vi "Dual_DM_Control_Main_V2.vi"(7 "Calling VI Ref":refnum<vi>) -> ()   [LabVIEW 2016]
uses:
  Controls/MirrorModes.ctl
  Hardware Configuration/Hardware Configuration Controls/Standard Action.ctl
  <vilib>/Utility/miscctls.llb/LVPointTypeDef.ctl
  <vilib>/Analysis/baseanly.llb/Mean (DBL).vi
  <vilib>/Utility/file.llb/Read Delimited Spreadsheet (DBL).vi
  <vilib>/Analysis/NI_AALBase.lvlib
  <vilib>/Utility/file.llb/Write To Spreadsheet File (DBL).vi
  <vilib>/Utility/file.llb/Read From Spreadsheet File (DBL).vi
panel:
  in  "Astig On/Off":bool
  in  "Load Astig":bool
  in  "Active Mirror":enum32{"Mirror 1", "Mirror 2"}(radio)
  in  "Clear Modes":bool
  in  "Mirror Modes":T1
  in  "Load Modes":bool
  in  "Save Modes":bool
  in  "Load Flat":bool
  in  "Apply Zero":bool
  in  "Load V Map":bool
  in  "Save V Map":bool
  in  "Apply Flat":bool
  in  "Center Bias":bool
  in  "Quit":bool
  out "Pixel Map (-1 to 1)":dbl[][](graph)
  # "Mode"
  # "Amount (nm)"
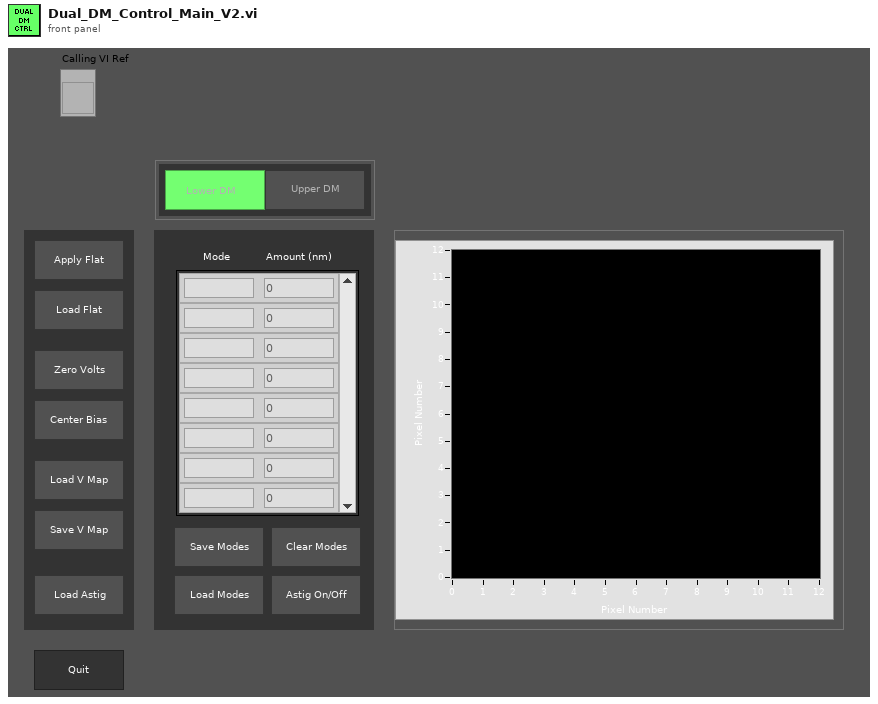
[diagram p1: front panel]
types:
  T1 = typedef "MirrorModes.ctl" = cluster{"Mode":string, "Amplitude":dbl}[]
  T2 = enum16{"Always On", "Always Off", "Off While Running"}
  T3 = typedef "LVPointTypeDef.ctl" = cluster{"Horizontal":i16, "Vertical":i16}
  T4 = typedef "Standard Action.ctl" = enum16{"Read", "Write"}
  T5 = typedef "MirrorModes_DUAL.ctl" = cluster{"Mode":string, "Amplitude":dbl}[][]
  T6 = typedef "LVRectTypeDef.ctl" = cluster{"Left":i16, "Top":i16, "Right":i16, "Bottom":i16}
  T7 = typedef "LVBoundsTypeDef.ctl" = cluster{"Width":u32, "Height":u32}
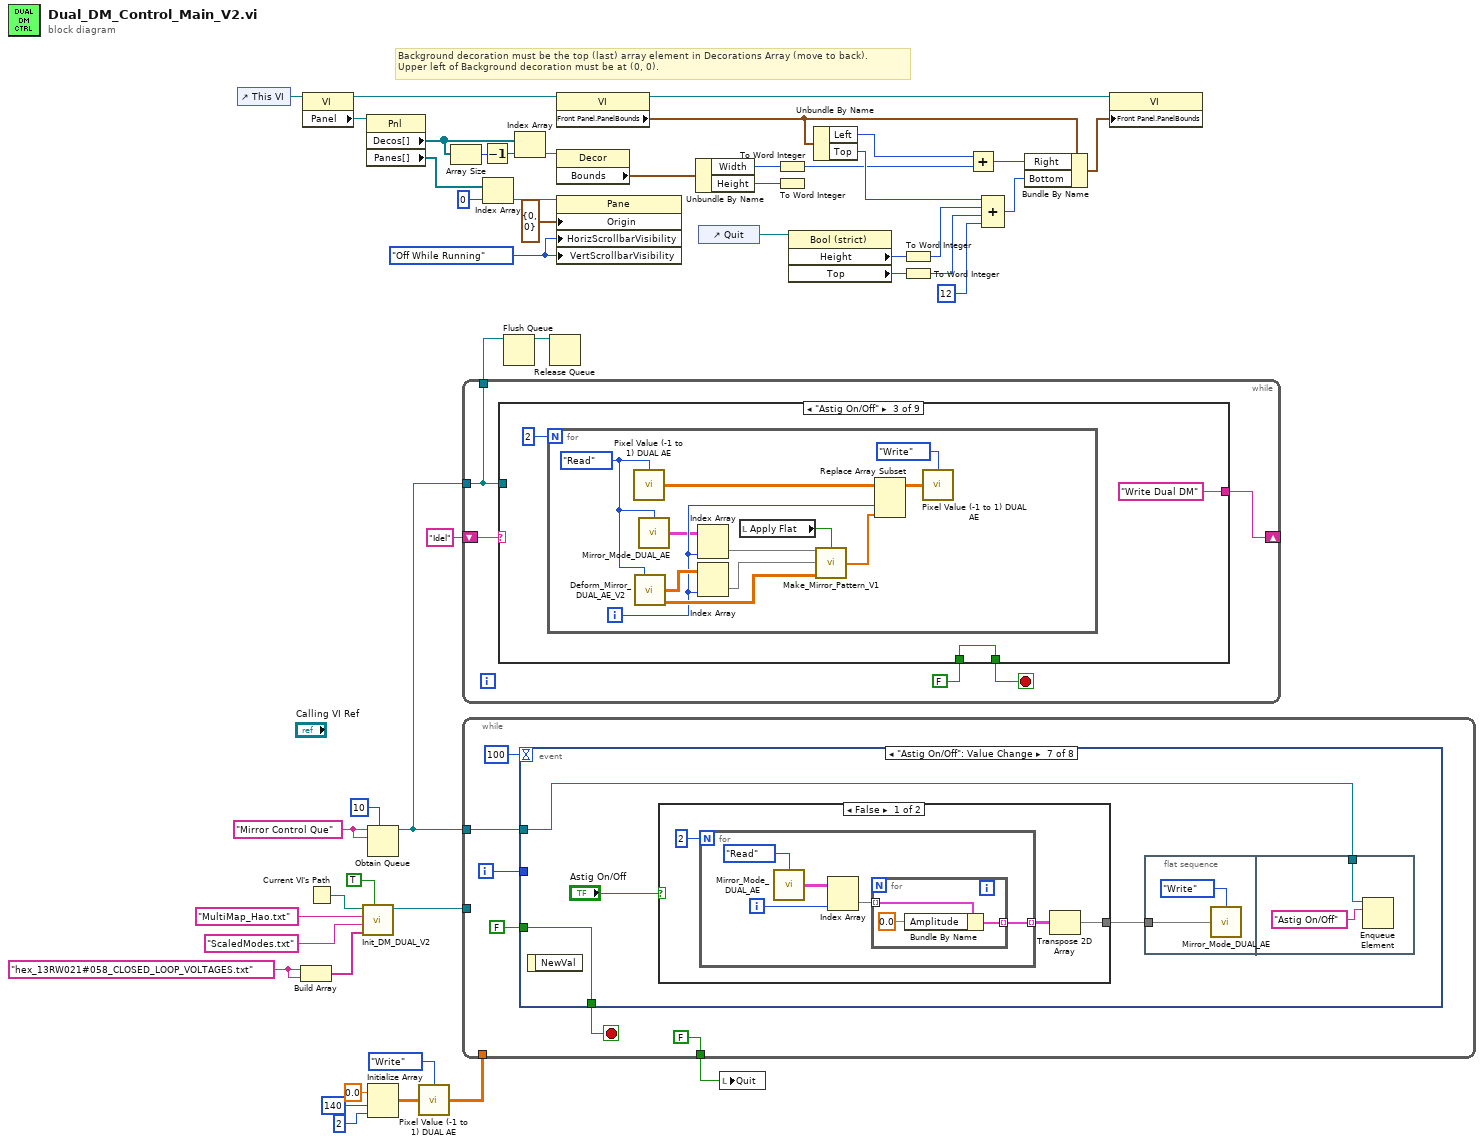
[diagram p0: block diagram]
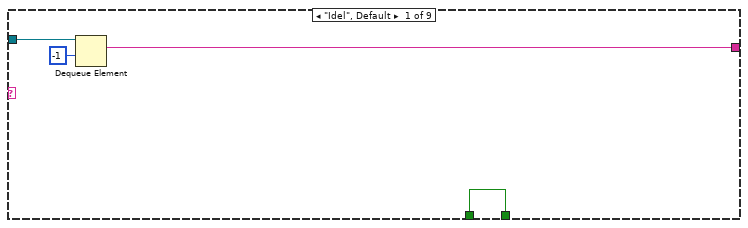
[diagram p2: hidden frame]
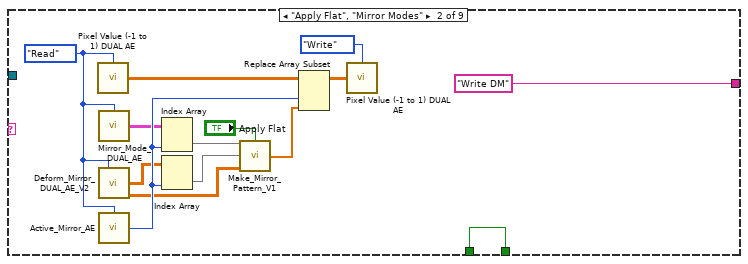
[diagram p3: hidden frame]
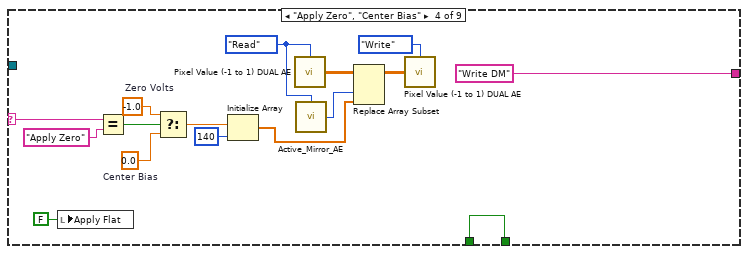
[diagram p4: hidden frame]
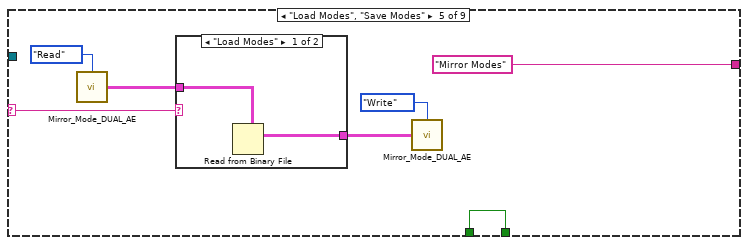
[diagram p5: hidden frame]
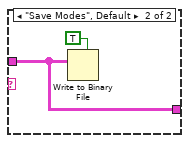
[diagram p6: hidden frame]
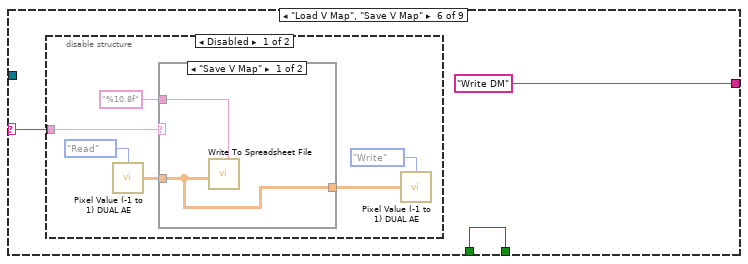
[diagram p7: hidden frame]
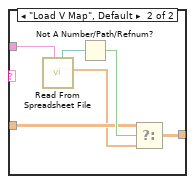
[diagram p8: hidden frame]
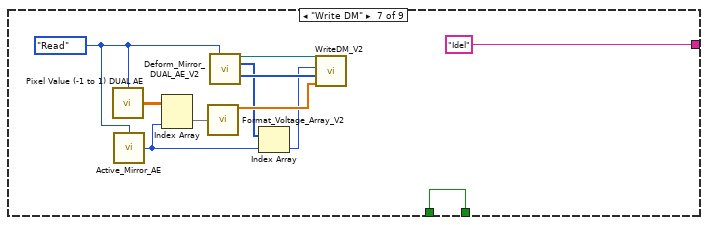
[diagram p10: hidden frame]
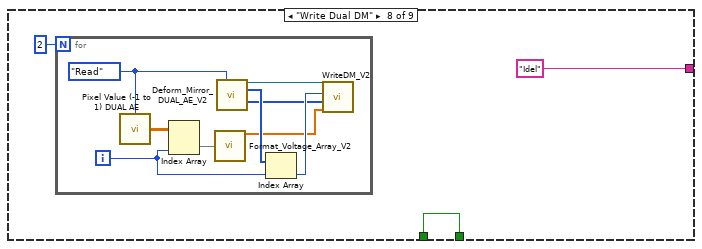
[diagram p11: hidden frame]
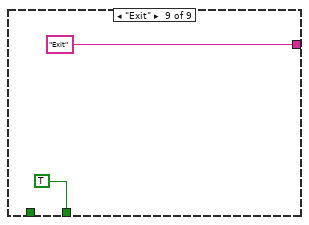
[diagram p12: hidden frame]
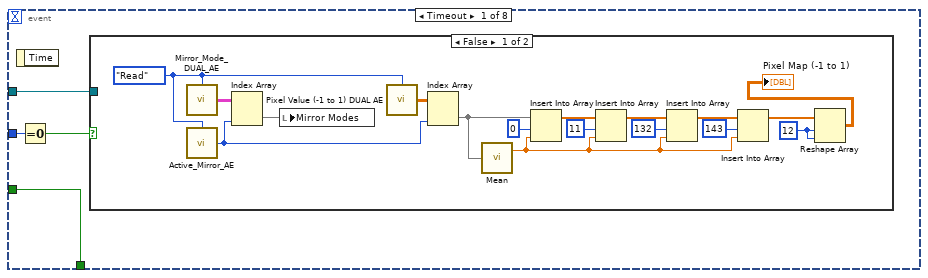
[diagram p13: hidden frame]
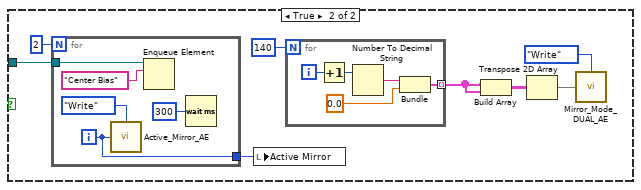
[diagram p14: hidden frame]
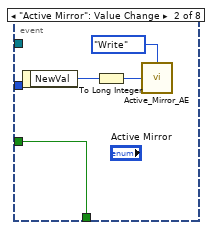
[diagram p15: hidden frame]
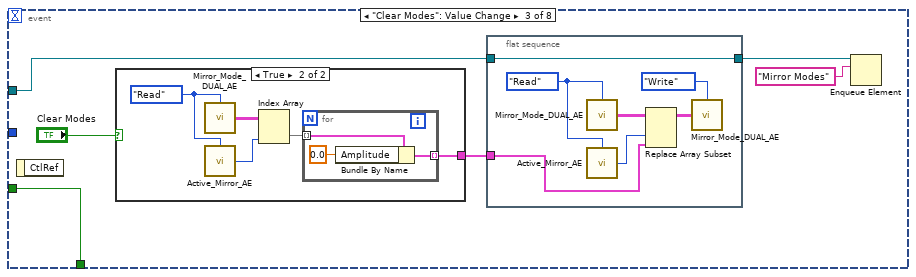
[diagram p16: hidden frame]
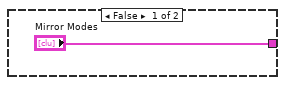
[diagram p17: hidden frame]
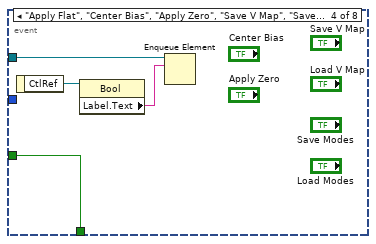
[diagram p18: hidden frame]
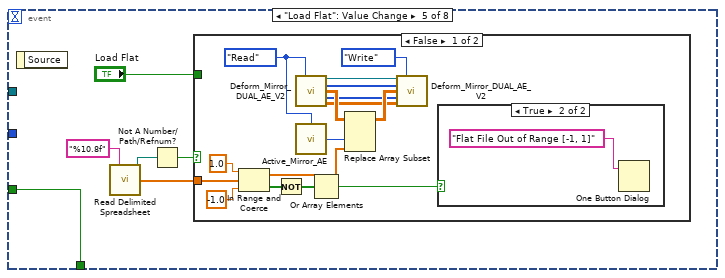
[diagram p19: hidden frame]
diagram:
  w13 = T2."Off While Running" ("Vertical Scrollbar Visibility")
  w38 = "hex_13RW021#058_CLOSED_LOOP_VOLTAGES.txt" ("name or relative path")
  w49 = "Mirror Control Que" ("name (unnamed)")
  # "Background decoration must be the top (last) array element in Decorations Array (move to back).\nUpper left of Background decoration must be at (0, 0)."
  n1 = control-ref of="This VI"() -> (w5:refnum<vi>)
  n2 = Build Array(w38, w38) -> (w37:string[])
  n3 = property class="VI"(reference=w5) -> (reference out=w14:refnum<vi>, "Panel"=w6:refnum<vi>)  [unwired: 1 in, 1 out]
  n4 = Current VI's Path() -> (path=w41:path)
  n5 = call "Init_DM_DUAL_V2.vi"("BM Flat"=TRUE, "BM Flat File"=w37, "Mirror Modes File"="ScaledModes.txt" ("name or relative path"), "DM Mapping File"="MultiMap_Hao.txt" ("name or relative path"), "Base File Path"=w41) -> ("reference out"=w47:refnum<k7>)  [unwired: 6 in]
  n6 = property class="Pnl"(reference=w6) -> ("Decos[]"=w4:refnum<vi>[], "Panes[]"=w10:refnum<vi>[])  [unwired: 1 in, 2 out]
  n7 = Obtain Queue(max queue size (-1, unlimited)=10, name (unnamed)=w49, element data type=w49) -> (queue out=w43:refnum<queue>)  [unwired: 2 in, 2 out]
  n8 = Initialize Array(0.0 ("element"), 140 ("dimension size"), 2 ("dimension size")) -> (w33:dbl[][])
  n9 = call "Pixel Value (-1 to 1) DUAL AE.vi"("Action"=Standard_Action."Write", "Pixel Value (-1 to 1)"=w33) -> ("Pixel Value (-1 to 1) Out"=w31:dbl[][])  [unwired: 13 in]
  n10 = Array Size(array=w4) -> (size(s)=w2:i32)
  n11 = while {
    tunnel: w43 -> [w50]
    shift-right: [w54] -> _
    shift-left: "Idel" ("name (unnamed)") -> [w53]
    tunnel: [w50] -> w46
    stop <- w52 stop-if-true
    n12 = case shown="\"Astig On/Off\"" w53 {
      selector: w53 -> [_ _ _ w99 w106 w116 _ _ _]
      tunnel: w50 -> [w58 _ _ _ _ _ _ _ _]
      tunnel: [w56 "Write DM" ("name (unnamed)") "Write Dual DM" ("name (unnamed)") "Write DM" ("name (unnamed)") "Mirror Modes" ("name (unnamed)") "Write DM" ("name (unnamed)") "Idel" ("name (unnamed)") "Idel" ("name (unnamed)") "Exit" ("name (unnamed)")] -> w54
      tunnel: [w55 w71 w74 w103 w110 w117 w142 w145 TRUE] -> w52
      tunnel: FALSE -> [w55 w71 w74 w103 w110 w117 w142 w145 _]
      frame "Idel", Default {
        n13 = Dequeue Element(queue=w58, timeout in ms (-1)=-1) -> (element=w56:string)  [unwired: 1 in, 3 out]
      }
      frame "Apply Flat", "Mirror Modes" {
        w66 = Standard_Action."Read" ("Action")
        n14 = call "Pixel Value (-1 to 1) DUAL AE.vi"("Action"=w66) -> ("Pixel Value (-1 to 1) Out"=w67:dbl[][])  [unwired: 14 in]
        n15 = call "Mirror_Mode_DUAL_AE.vi"("Action"=w66) -> ("Mirror Modes Out"=w63:T5)  [unwired: 14 in]
        n16 = call "Deform_Mirror_DUAL_AE_V2.vi"("Action"=w66) -> ("Flat Files Out"=w61:dbl[][], "Mode Matrix Out"=w60:dbl[][])  [unwired: 10 in, 3 out]
        n17 = call "Active_Mirror_AE.vi"("Action"=w66) -> ("Active Mirror"=w69:i32)  [unwired: 14 in]
        n18 = Index Array(array=w63, index (col)=w69) -> (element=w64:cluster{"Mode":string, "Amplitude":dbl}[])  [unwired: 1 in]
        n19 = Index Array(array=w61, index (col)=w69) -> (element=w62:dbl[])  [unwired: 1 in]
        n20 = call "Make_Mirror_Pattern_V1.vi"("Mirror Modes In"=w64, "Flat On?"="Apply Flat", "Flat File In"=w62, "Mirror Modes Array"=w60) -> ("Pixel Value U (-1 to 1)"=w68:dbl[])  [unwired: 11 in]
        n21 = Replace Array Subset(array=w67, new element=w68, index (col)=w69) -> (w70:dbl[][])  [unwired: 1 in]
        n22 = call "Pixel Value (-1 to 1) DUAL AE.vi"("Action"=Standard_Action."Write", "Pixel Value (-1 to 1)"=w70) -> ()  [unwired: 13 in, 1 out]
      }
      frame "Astig On/Off" {
        n23 = for {
          N: 2 -> [_]
          i -> [w78]
          w76 = Standard_Action."Read" ("Action")
          n24 = call "Pixel Value (-1 to 1) DUAL AE.vi"("Action"=w76) -> ("Pixel Value (-1 to 1) Out"=w82:dbl[][])  [unwired: 14 in]
          n25 = call "Deform_Mirror_DUAL_AE_V2.vi"("Action"=w76) -> ("Flat Files Out"=w86:dbl[][], "Mode Matrix Out"=w87:dbl[][])  [unwired: 10 in, 3 out]
          n26 = call "Mirror_Mode_DUAL_AE.vi"("Action"=w76) -> ("Mirror Modes Out"=w77:T5)  [unwired: 14 in]
          n27 = Index Array(array=w77, index (col)=w78) -> (element=w84:cluster{"Mode":string, "Amplitude":dbl}[])  [unwired: 1 in]
          n28 = Index Array(array=w86, index (col)=w78) -> (element=w85:dbl[])  [unwired: 1 in]
          n29 = local read "Apply Flat"() -> (w79:bool)
          n30 = call "Make_Mirror_Pattern_V1.vi"("Mirror Modes In"=w84, "Flat On?"=w79, "Flat File In"=w85, "Mirror Modes Array"=w87) -> ("Pixel Value U (-1 to 1)"=w81:dbl[])  [unwired: 11 in]
          n31 = Replace Array Subset(array=w82, new element=w81, index (col)=w78) -> (w80:dbl[][])  [unwired: 1 in]
          n32 = call "Pixel Value (-1 to 1) DUAL AE.vi"("Action"=Standard_Action."Write", "Pixel Value (-1 to 1)"=w80) -> ()  [unwired: 13 in, 1 out]
        }
      }
      frame "Apply Zero", "Center Bias" {
        w91 = Standard_Action."Read" ("Action")
        w95 = -1.0  # Zero Volts
        w97 = 0.0  # Center Bias
        n33 = local write "Apply Flat"(FALSE ("Apply Flat")) -> ()
        n34 = Equal?(x=w99, y="Apply Zero") -> (x = y?=w98:bool)
        n35 = Select(t=w95, s=w98, f=w97) -> (s? t:f=w96:dbl)
        n36 = Initialize Array(w96, 140 ("dimension size")) -> (w88:dbl[])
        n37 = call "Pixel Value (-1 to 1) DUAL AE.vi"("Action"=w91) -> ("Pixel Value (-1 to 1) Out"=w89:dbl[][])  [unwired: 14 in]
        n38 = call "Active_Mirror_AE.vi"("Action"=w91) -> ("Active Mirror"=w90:i32)  [unwired: 14 in]
        n39 = Replace Array Subset(array=w89, new element=w88, index (col)=w90) -> (w93:dbl[][])  [unwired: 1 in]
        n40 = call "Pixel Value (-1 to 1) DUAL AE.vi"("Action"=Standard_Action."Write", "Pixel Value (-1 to 1)"=w93) -> ()  [unwired: 13 in, 1 out]
      }
      frame "Load Modes", "Save Modes" {
        n41 = call "Mirror_Mode_DUAL_AE.vi"("Action"=Standard_Action."Read") -> ("Mirror Modes Out"=w105:T5)  [unwired: 14 in]
        n42 = case shown="\"Load Modes\"" w106 {
          tunnel: w105 -> [w112 w113]
          tunnel: [w111 w113] -> w104
          frame "Load Modes" {
            n43 = Read from Binary File(5:w112) -> (2:w111:T5)  [unwired: 5 in, 3 out]
          }
          frame "Save Modes", Default {
            n44 = Write to Binary File(data=w113, 5:TRUE ("prepend array or string size? (T)")) -> ()  [unwired: 4 in, 3 out]
          }
        }
        n45 = call "Mirror_Mode_DUAL_AE.vi"("Action"=Standard_Action."Write", "Mirror Modes In"=w104) -> ()  [unwired: 13 in, 1 out]
      }
      frame "Load V Map", "Save V Map" {
        n46 = disable-structure shown="Disabled" {
          disable-tunnel: w116 -> [w123 _]
          frame Disabled {
            n47 = call "Pixel Value (-1 to 1) DUAL AE.vi"("Action"=Standard_Action."Read") -> ("Pixel Value (-1 to 1) Out"=w121:dbl[][])  [unwired: 14 in]
            n48 = case shown="\"Save V Map\"" w123 {
              tunnel: w121 -> [w124 w128]
              tunnel: "%10.8f" -> [w125 w131]
              tunnel: [w124 w126] -> w118
              frame "Save V Map" {
                n49 = call-poly <vilib>:"Write To Spreadsheet File.vi"("format (%.3f)"=w125, "1D data"=w124) -> ()  [unwired: 6 in, 1 out]
              }
              frame "Load V Map", Default {
                n50 = call-poly <vilib>:"Read From Spreadsheet File.vi"("format (%.3f)"=w131) -> ("first row"=w127:dbl[], "new file path (Not A Path if cancelled)"=w130:path)  [unwired: 6 in, 3 out]
                n51 = Not A Number/Path/Refnum?(number/path/refnum=w130) -> (NaN/Path/Refnum?=w129:bool)
                n52 = Select(t=w128, s=w129, f=w127) -> (s? t:f=w126:dbl[][])
              }
            }
            n53 = call "Pixel Value (-1 to 1) DUAL AE.vi"("Action"=Standard_Action."Write", "Pixel Value (-1 to 1)"=w118) -> ()  [unwired: 13 in, 1 out]
          }
          frame Enabled {
          }
        }
      }
      frame "Write DM" {
        w135 = Standard_Action."Read" ("Action")
        n54 = call "Pixel Value (-1 to 1) DUAL AE.vi"("Action"=w135) -> ("Pixel Value (-1 to 1) Out"=w137:dbl[][])  [unwired: 14 in]
        n55 = call "Active_Mirror_AE.vi"("Action"=w135) -> ("Active Mirror"=w133:i32)  [unwired: 14 in]
        n56 = Index Array(array=w137, index (col)=w133) -> (element=w136:dbl[])  [unwired: 1 in]
        n57 = call "Format_Voltage_Array_V2.vi"("Pixel Level (-1 to 1)"=w136) -> ("Voltage Array (Volts)"=w138:dbl[])  [unwired: 13 in, 1 out]
        n58 = call "Deform_Mirror_DUAL_AE_V2.vi"("Action"=w135) -> ("Refnum Out"=w140:refnum<k7>, "IDs Out"=w134:i32[], "Multi Map Data Out"=w139:i32[])  [unwired: 10 in, 2 out]
        n59 = Index Array(array=w134, index=w133) -> (element=w132:i32)
        n60 = call "WriteDM_V2.vi"("reference in"=w140, "nDevId"=w132, "MultiDM  Mapping"=w139, "Voltage Array in"=w138) -> ()  [unwired: 2 in, 2 out]
      }
      frame "Write Dual DM" {
        n61 = for {
          N: 2 -> [_]
          i -> [w146]
          w152 = Standard_Action."Read" ("Action")
          n62 = call "Pixel Value (-1 to 1) DUAL AE.vi"("Action"=w152) -> ("Pixel Value (-1 to 1) Out"=w150:dbl[][])  [unwired: 14 in]
          n63 = Index Array(array=w150, index (col)=w146) -> (element=w151:dbl[])  [unwired: 1 in]
          n64 = call "Format_Voltage_Array_V2.vi"("Pixel Level (-1 to 1)"=w151) -> ("Voltage Array (Volts)"=w149:dbl[])  [unwired: 13 in, 1 out]
          n65 = call "Deform_Mirror_DUAL_AE_V2.vi"("Action"=w152) -> ("Refnum Out"=w147:refnum<k7>, "IDs Out"=w153:i32[], "Multi Map Data Out"=w148:i32[])  [unwired: 10 in, 2 out]
          n66 = Index Array(array=w153, index=w146) -> (element=w154:i32)
          n67 = call "WriteDM_V2.vi"("reference in"=w147, "nDevId"=w154, "MultiDM  Mapping"=w148, "Voltage Array in"=w149) -> ()  [unwired: 2 in, 2 out]
        }
      }
      frame "Exit" {
      }
    }
  }
  n68 = while {
    tunnel: w43 -> [w158]
    tunnel: w47 -> [_]
    tunnel: w31 -> [_]
    tunnel: [FALSE] -> w1
    i -> [w159]
    stop <- w162 stop-if-true
    n69 = event shown="[6] \"Astig On/Off\": Value Change" {
      selector: _ -> [_ _ _ _ _ _ _ _]
      dyn-events: _ -> [_ _ _ _ _ _ _ _]
      timeout: 100 -> [_ _ _ _ _ _ _ _]
      tunnel: [w166 w205 w211 w231 w237 w259 w263 w292] -> w162
      tunnel: FALSE -> [w166 w205 w211 w231 w237 w259 w263 _]
      tunnel: w159 -> [w165 _ _ _ _ _ _ _]
      tunnel: w158 -> [w163 _ w210 w230 _ _ w260 w290]
      event Timeout {
        n70 = event-data() -> ()  [unwired: 1 in, 1 out]
        n71 = Equal To 0?(x=w165) -> (x = 0?=w164:bool)
        n72 = case shown="False" w164 {
          tunnel: w163 -> [_ w191]
          frame False {
            w179 = 12 ("dimension size")
            w180 = Standard_Action."Read" ("Action")
            n73 = call "Mirror_Mode_DUAL_AE.vi"("Action"=w180) -> ("Mirror Modes Out"=w167:T5)  [unwired: 14 in]
            n74 = call "Active_Mirror_AE.vi"("Action"=w180) -> ("Active Mirror"=w182:i32)  [unwired: 14 in]
            n75 = Index Array(array=w167, index (col)=w182) -> (element=w168:cluster{"Mode":string, "Amplitude":dbl}[])  [unwired: 1 in]
            n76 = local write "Mirror Modes"(w168) -> ()
            n77 = call "Pixel Value (-1 to 1) DUAL AE.vi"("Action"=w180) -> ("Pixel Value (-1 to 1) Out"=w181:dbl[][])  [unwired: 14 in]
            n78 = Index Array(array=w181, index (col)=w182) -> (element=w183:dbl[])  [unwired: 1 in]
            n79 = call-poly <vilib>:"Mean.vi"("X"=w183) -> ("mean"=w177:dbl)  [unwired: 1 out]
            n80 = Insert Into Array(array=w183, index=0, new element=w177) -> (w172:dbl[])
            n81 = Insert Into Array(array=w172, index=11, new element=w177) -> (w174:dbl[])
            n82 = Insert Into Array(array=w174, index=132, new element=w177) -> (w176:dbl[])
            n83 = Insert Into Array(array=w176, index=143, new element=w177) -> (w169:dbl[])
            n84 = Reshape Array(w169, w179, w179) -> (→"Pixel Map (-1 to 1)":dbl[][])
          }
          frame True {
            n85 = for {
              N: 2 -> [_]
              tunnel: w191 -> [w196]
              tunnel: [w192] -> w184
              i -> [w192]
              n86 = call "Active_Mirror_AE.vi"("Action"=Standard_Action."Write", "Active Mirror In"=w192) -> ()  [unwired: 13 in, 1 out]
              n87 = Enqueue Element(queue=w196, element="Center Bias") -> ()  [unwired: 2 in, 3 out]
              n88 = Wait (ms)(milliseconds to wait=u32 300) -> ()  [unwired: 1 out]
            }
            n89 = local write "Active Mirror"(w184) -> ()
            n90 = for {
              N: 140 -> [_]
              tunnel: [w197] -> w188 mode=indexing
              i -> [w201]
              n91 = Increment(x=w201) -> (x+1=w200:i32)
              n92 = Number To Decimal String(number=w200) -> (decimal integer string=w199:string)  [unwired: 1 in]
              n93 = Bundle(w199, 0.0) -> (w197:cluster{string, dbl})  [unwired: 1 in]
            }
            n94 = Build Array(w188, w188) -> (w186:cluster{string, dbl}[][])
            n95 = Transpose 2D Array(2D array=w186) -> (transposed array=w185:cluster{string, dbl}[][])
            n96 = call "Mirror_Mode_DUAL_AE.vi"("Action"=Standard_Action."Write", "Mirror Modes In"=w185) -> ()  [unwired: 13 in, 1 out]
          }
        }
      }
      event "Active Mirror": Value Change {
        n97 = event-data() -> ("NewVal"=w204:enum32{"Mirror 1", "Mirror 2"})  [unwired: 1 in]
        n98 = To Long Integer(number=w204) -> (32bit integer=w203:i32)
        n99 = call "Active_Mirror_AE.vi"("Action"=Standard_Action."Write", "Active Mirror In"=w203) -> ()  [unwired: 13 in, 1 out]
      }
      event "Clear Modes": Value Change {
        n100 = event-data() -> ()  [unwired: 1 in, 1 out]
        n101 = case shown="True" "Clear Modes" {
          tunnel: ["Mirror Modes" w213] -> w206
          frame False {
          }
          frame True {
            w216 = Standard_Action."Read" ("Action")
            n102 = call "Mirror_Mode_DUAL_AE.vi"("Action"=w216) -> ("Mirror Modes Out"=w215:T5)  [unwired: 14 in]
            n103 = call "Active_Mirror_AE.vi"("Action"=w216) -> ("Active Mirror"=w217:i32)  [unwired: 14 in]
            n104 = Index Array(array=w215, index (col)=w217) -> (element=w214:cluster{"Mode":string, "Amplitude":dbl}[])  [unwired: 1 in]
            n105 = for {
              tunnel: w214 -> [w220] mode=indexing
              tunnel: [w218] -> w213 mode=indexing
              n106 = Bundle By Name(cluster=w220, "Amplitude"=0.0) -> (w218:cluster{"Mode":string, "Amplitude":dbl})
            }
          }
        }
        n107 = flat-sequence {
          tunnel: w206 -> [w221]
          tunnel: w210 -> [w227]
          tunnel: [w227] -> w208
          frame #0 {
            w224 = Standard_Action."Read" ("Action")
            n108 = call "Mirror_Mode_DUAL_AE.vi"("Action"=w224) -> ("Mirror Modes Out"=w223:T5)  [unwired: 14 in]
            n109 = call "Active_Mirror_AE.vi"("Action"=w224) -> ("Active Mirror"=w225:i32)  [unwired: 14 in]
            n110 = Replace Array Subset(array=w223, new element=w221, index (col)=w225) -> (w226:T5)  [unwired: 1 in]
            n111 = call "Mirror_Mode_DUAL_AE.vi"("Action"=Standard_Action."Write", "Mirror Modes In"=w226) -> ()  [unwired: 13 in, 1 out]
          }
        }
        n112 = Enqueue Element(queue=w208, element="Mirror Modes") -> ()  [unwired: 2 in, 3 out]
      }
      event "Apply Flat", "Center Bias", "Apply Zero", "Save V Map", "Save Modes", "Load Modes", "Load V Map": Value Change {
        n113 = event-data() -> ("CtlRef"=w229:refnum<vi>)  [unwired: 1 in]
        n114 = property class="Bool"(reference=w229) -> ("Label.Text"=w228:string)  [unwired: 1 in, 2 out]
        n115 = Enqueue Element(queue=w230, element=w228) -> ()  [unwired: 2 in, 3 out]
      }
      event "Load Flat": Value Change {
        n116 = event-data() -> ()  [unwired: 1 in, 1 out]
        n117 = call-poly <vilib>:"Read Delimited Spreadsheet.vi"("format (%.3f)"="%10.8f") -> ("new file path (Not A Path if cancelled)"=w235:path, "first row"=w233:dbl[])  [unwired: 9 in, 4 out]
        n118 = Not A Number/Path/Refnum?(number/path/refnum=w235) -> (NaN/Path/Refnum?=w234:bool)
        n119 = case shown="False" w234 {
          tunnel: w233 -> [w253 _]
          tunnel: "Load Flat" -> [_ _]
          frame False {
            w244 = Standard_Action."Read" ("Action")
            n120 = In Range and Coerce(upper limit=1.0, x=w253, lower limit=-1.0) -> (coerced(x)=w238:dbl[], In Range?=w250:bool[])
            n121 = Not(x=w250) -> (.not. x?=w249:bool[])
            n122 = call "Deform_Mirror_DUAL_AE_V2.vi"("Action"=w244) -> ("Refnum Out"=w239:refnum<k7>, "IDs Out"=w240:i32[], "Flat Files Out"=w245:dbl[][], "Multi Map Data Out"=w241:i32[], "Mode Matrix Out"=w242:dbl[][])  [unwired: 10 in]
            n123 = call "Active_Mirror_AE.vi"("Action"=w244) -> ("Active Mirror"=w247:i32)  [unwired: 14 in]
            n124 = Or Array Elements(Boolean array=w249) -> (logical OR=w248:bool)
            n125 = Replace Array Subset(array=w245, new element=w238, index (col)=w247) -> (w246:dbl[][])  [unwired: 1 in]
            n126 = call "Deform_Mirror_DUAL_AE_V2.vi"("Refnum In"=w239, "Action"=Standard_Action."Write", "IDs In"=w240, "Flat Files In"=w246, "Multi Map Data In"=w241, "Mode Matrix"=w242) -> ()  [unwired: 5 in, 5 out]
            n127 = case shown="True" w248 {
              frame False {
              }
              frame True {
                n128 = One Button Dialog(message="Flat File Out of Range [-1, 1]") -> ()  [unwired: 1 in, 1 out]
              }
            }
          }
          frame True {
          }
        }
      }
      event "Load Astig": Value Change {
        n129 = event-data() -> ()  [unwired: 1 in, 1 out]
        n130 = call "Astig Modes AE.vi"("Action"=Standard_Action."Read") -> ("Mirror Modes Out"=w258:T5)  [unwired: 14 in]
        n131 = Read from Binary File(5:w258) -> (2:w255:T5)  [unwired: 5 in, 3 out]
        n132 = call "Astig Modes AE.vi"("Action"=Standard_Action."Write", "Mirror Modes In"=w255) -> ()  [unwired: 13 in, 1 out]
      }
      event "Astig On/Off": Value Change {
        n133 = event-data() -> ()  [unwired: 1 in, 1 out]
        n134 = case shown="False" "Astig On/Off" {
          tunnel: [w268 w280] -> w261
          frame False {
            n135 = for {
              N: 2 -> [_]
              tunnel: [w271] -> w269 mode=indexing
              i -> [w272]
              n136 = call "Mirror_Mode_DUAL_AE.vi"("Action"=Standard_Action."Read") -> ("Mirror Modes Out"=w274:T5)  [unwired: 14 in]
              n137 = Index Array(array=w274, index (col)=w272) -> (element=w275:cluster{"Mode":string, "Amplitude":dbl}[])  [unwired: 1 in]
              n138 = for {
                tunnel: w275 -> [w278] mode=indexing
                tunnel: [w276] -> w271 mode=indexing
                n139 = Bundle By Name(cluster=w278, "Amplitude"=0.0) -> (w276:cluster{"Mode":string, "Amplitude":dbl})
              }
            }
            n140 = Transpose 2D Array(2D array=w269) -> (transposed array=w268:cluster{"Mode":string, "Amplitude":dbl}[][])
          }
          frame True {
            n141 = call "Astig Modes AE.vi"("Action"=Standard_Action."Read") -> ("Mirror Modes Out"=w280:T5)  [unwired: 14 in]
          }
        }
        n142 = flat-sequence {
          tunnel: w261 -> [w265]
          tunnel: w260 -> [w266]
          frame #0 {
            n143 = call "Mirror_Mode_DUAL_AE.vi"("Action"=Standard_Action."Write", "Mirror Modes In"=w265) -> ()  [unwired: 13 in, 1 out]
          }
          frame #1 {
            n144 = Enqueue Element(queue=w266, element="Astig On/Off") -> ()  [unwired: 2 in, 3 out]
          }
        }
      }
      event "Quit": Value Change {
        n145 = event-data() -> ("NewVal"=w292:bool)  [unwired: 1 in]
        n146 = for {
          N: 2 -> [_]
          tunnel: w290 -> [w298]
          tunnel: [w293] -> w281
          i -> [w294]
          n147 = call "Active_Mirror_AE.vi"("Action"=Standard_Action."Write", "Active Mirror In"=w294) -> ()  [unwired: 13 in, 1 out]
          n148 = Enqueue Element(queue=w298, element="Apply Zero") -> (queue out=w293:refnum<queue>)  [unwired: 2 in, 2 out]
          n149 = Wait (ms)(milliseconds to wait=u32 300) -> ()  [unwired: 1 out]
        }
        n150 = Enqueue Element(queue=w281, element="Exit") -> (error out=w285:errorcluster)  [unwired: 2 in, 2 out]
        n151 = call "Deform_Mirror_DUAL_AE_V2.vi"("Action"=Standard_Action."Read") -> ("Refnum Out"=w288:refnum<k7>, "IDs Out"=w283:i32[])  [unwired: 10 in, 3 out]
        n152 = call "ConfigDM.vi"("High Voltage"=FALSE, "error in (no error)"=w285, "Dev IDs"=w283, "Automation Refnum in"=w288) -> ("error out"=w284:errorcluster, "Automation Refnum out"=w287:refnum<k7>)  [unwired: 6 in]
        n153 = Close Reference(reference=w287, error in (no error)=w284) -> ()  [unwired: 1 out]
      }
    }
  }
  n154 = Decrement(x=w2) -> (x-1=w3:i32)
  n155 = Index Array(array=w10, index=0) -> (element=w9:refnum<vi>)
  n156 = Flush Queue(queue=w46) -> (queue out=w45:refnum<queue>)  [unwired: 1 in, 2 out]
  n157 = Index Array(array=w4, index=w3) -> (element=w12:refnum<vi>)
  n158 = Release Queue(queue=w45) -> ()  [unwired: 2 in, 3 out]
  n159 = property class="VI"(reference=w14) -> (reference out=w16:refnum<vi>, "Front Panel.PanelBounds"=w17:T6)  [unwired: 1 in, 1 out]
  n160 = property class="Decor"(reference=w12) -> ("Bounds"=w15:T7)  [unwired: 1 in, 2 out]
  n161 = property class="Pane"(reference=w9, "Origin"=T3 {"Horizontal"=0, "Vertical"=0}, "HorizScrollbarVisibility"=w13, "VertScrollbarVisibility"=w13) -> ()  [unwired: 1 in, 2 out]
  n162 = Unbundle By Name(w15) -> ("Width"=w20:u32, "Height"=w23:u32)
  n163 = control-ref of="Quit"() -> (w7:refnum<vi>)
  n164 = local write "Quit"(w1) -> ()
  n165 = To Word Integer(number=w20) -> (16bit integer=w22:i16)
  n166 = To Word Integer(number=w23) -> ()  [unwired: 1 out]
  n167 = property class="Bool (strict)"(reference=w7) -> ("Height"=w25:u32, "Top"=w26:i32)  [unwired: 1 in, 2 out]
  n168 = Unbundle By Name(w17) -> ("Left"=w19:i16, "Top"=w30:i16)
  n169 = To Word Integer(number=w25) -> (16bit integer=w28:i16)
  n170 = To Word Integer(number=w26) -> (16bit integer=w29:i16)
  n171 = Add(x=w19, y=w22) -> (x+y=w21:i16)
  n172 = Compound Arithmetic op=ADD(w30, w28, w29, i16 12 ("y")) -> (w24:i16)
  n173 = Bundle By Name(cluster=w17, "Right"=w21, "Bottom"=w24) -> (w18:T6)
  n174 = property class="VI"(reference=w16, "Front Panel.PanelBounds"=w18) -> ()  [unwired: 1 in, 2 out]
